vi "Settings.vi"(8 "error in (no error)":errorcluster, 9 "Region":i32=3, 11 "Workspace in":refnum<class "Fixture.lvclass">) -> (0 "error out":errorcluster, 3 "Workspace out":refnum<class "Fixture.lvclass">)   [LabVIEW 2016, in "Fixture.lvclass"]
uses:
  Fixture.lvclass
  Fixture.lvclass/Fixture.ctl
panel:
  in  "Position":i32=4
  in  "Submit":bool
  # "Pick Up Tool"
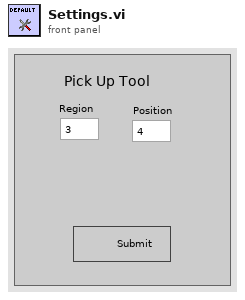
[diagram p1: front panel]
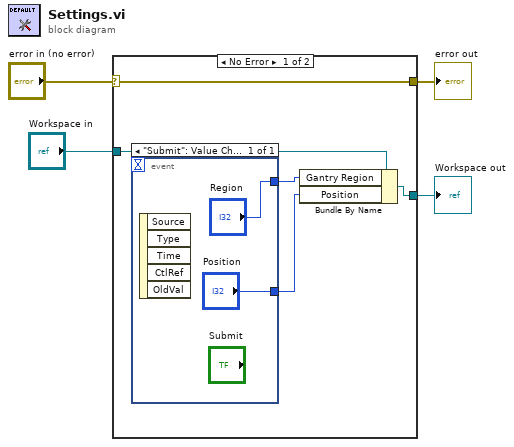
[diagram p0: block diagram]
diagram:
  n1 = case shown="No Error" "error in (no error)" {
    selector: "error in (no error)" -> [w9 w13]
    tunnel: [w9 w13] -> w3
    tunnel: [w7 w12] -> w1
    tunnel: "Workspace in" -> [w8 w12]
    frame No Error {
      n2 = event shown="[0] \"Submit\": Value Change" {
        selector: _ -> [_]
        dyn-events: _ -> [_]
        timeout: _ -> [_]
        tunnel: ["Region"] -> w6
        tunnel: ["Position"] -> w5
        event "Submit": Value Change {
          n3 = event-data() -> ()  [unwired: 1 in, 5 out]
        }
      }
      n4 = Bundle By Name(cluster=w8, "Gantry Region"=w6, "Position"=w5) -> (w7:refnum<class "Fixture.lvclass">)
    }
    frame Error {
    }
  }
  "error out" <- w3
  "Workspace out" <- w1
